vi "rszvl_core_global.vi"() -> ()   [LabVIEW 2014] (continued)
 on the Y axis, the entered numerical values are dimensionless.\n\nAvailable Repeated Capabilities:\nNone\n\nRemote-control command(s):\nCALCulate:STATistics:SCALe:Y:UPPer", "Flags"={"OPC Wait"=FALSE, "Dont check status"=FALSE, "*WAI"=FALSE}, "Check Status Callback"=""}, {"Level"=3, "Descriptive Name"="Signal Statistic Adjust Settings", "Class Only"=FALSE, "Data Type"=4, "Access"=1, "Identifier"="RSZVL_ATTR_MEAS_STAT_ADJ", "Range Table"="", "Command"="CALC:STAT:SCAL:AUTO ONCE", "Read Callback"="", "Write Callback"="", "Range Callback"="", "Check Callback"="", "Rngtable Callback"="", "Coerce Callback"="", "User Callback"="", "Supported Models"="", "Instrument Options"="", "Repeated Capabilities"="", "Restricted Repeated Capabilities"="", "Help"="This attribute optimizes the level setting of the instrument depending on the measured peak power, in order to obtain maximum instrument sensitivity.\nTo obtain maximum resolution, the level range is set as a function of the measured spacing between peak power and the minimum power for the APD measurement and of the spacing between peak power and mean power for the CCDF measurement. In addition, the probability scale for the number of test points is adapted.\n\nAvailable Repeated Capabilities:\nNone\n\nRemote-control command(s):\nCALCulate:STATistics:SCALe:AUTO ONCE", "Flags"={"OPC Wait"=TRUE, "Dont check status"=FALSE, "*WAI"=FALSE}, "Check Status Callback"=""}, {"Level"=3, "Descriptive Name"="Signal Statistic Default Setting", "Class Only"=FALSE, "Data Type"=4, "Access"=1, "Identifier"="RSZVL_ATTR_MEAS_STAT_PRESET", "Range Table"="", "Command"="CALC:STAT:PRES", "Read Callback"="", "Write Callback"="", "Range Callback"="", "Check Callback"="", "Rngtable Callback"="", "Coerce Callback"="", "User Callback"="", "Supported Models"="", "Instrument Options"="", "Repeated Capabilities"="", "Restricted Repeated Capabilities"="", "Help"="This attribute resets the scaling of the X and Y axes in a statistical measurement. The following values are set:\nX axis ref level: -20 dBm\nX axis range APD: 100 dB\nX axis range CCDF: 20 dB\nY axis upper limit: 1.0\nY axis lower limit: 1E-6\n\nAvailable Repeated Capabilities:\nNone\n\nRemote-control command(s):\nCALCulate:STATistics:PRESet", "Flags"={"OPC Wait"=FALSE, "Dont check status"=FALSE, "*WAI"=FALSE}, "Check Status Callback"=""}, {"Level"=3, "Descriptive Name"="Signal Statistic Result", "Class Only"=FALSE, "Data Type"=1, "Access"=0, "Identifier"="RSZVL_ATTR_STAT_RESULT", "Range Table"="", "Command"="CALC:STAT:RES{Trace}? {StatisticMeasType}", "Read Callback"="", "Write Callback"="", "Range Callback"="", "Check Callback"="", "Rngtable Callback"="", "Coerce Callback"="", "User Callback"="", "Supported Models"="", "Instrument Options"="", "Repeated Capabilities"="", "Restricted Repeated Capabilities"="", "Help"="This attribute reads out the results of statistical measurements of a recorded trace.\n\nAvailable Repeated Capabilities:\nTrace: TR1,TR2,TR3,TR4,TR5,TR6,TR7,TR8,TR9,TR10,TR11,TR12,TR13,TR14,TR15,TR16,TR17,TR18,TR19,TR20\r\nStatisticMeasType: StatMean,StatPeak,StatCrestFactor\r\n\nRemote-control command(s):\nCALCulate:STATistics:RESult<1 to 3>? MEAN | PEAK | CFACtor", "Flags"={"OPC Wait"=FALSE, "Dont check status"=FALSE, "*WAI"=FALSE}, "Check Status Callback"=""}, {"Level"=2, "Descriptive Name"="Modulation Depth", "Class Only"=TRUE, "Data Type"=0, "Access"=0, "Identifier"="", "Range Table"="", "Command"="", "Read Callback"="", "Write Callback"="", "Range Callback"="", "Check Callback"="", "Rngtable Callback"="", "Coerce Callback"="", "User Callback"="", "Supported Models"="", "Instrument Options"="", "Repeated Capabilities"="", "Restricted Repeated Capabilities"="", "Help"="Modulation Depth measurement configuration and results.", "Flags"={"OPC Wait"=FALSE, "Dont check status"=FALSE, "*WAI"=FALSE}, "Check Status Callback"=""}, {"Level"=3, "Descriptive Name"="Modulation Depth State", "Class Only"=FALSE, "Data Type"=3, "Access"=2, "Identifier"="RSZVL_ATTR_MEAS_MDEPTH_STATE", "Range Table"="", "Command"="CALC:MARK:FUNC:MDEP", "Read Callback"="", "Write Callback"="", "Range Callback"="", "Check Callback"="", "Rngtable Callback"="", "Coerce Callback"="", "User Callback"="", "Supported Models"="", "Instrument Options"="", "Repeated Capabilities"="", "Restricted Repeated Capabilities"="", "Help"="This attribute switches on the measurement of the AM modulation depth. An AM-modulated carrier is required on the screen for correct operation. If necessary, marker 1 is previously activated and set to the largest signal available.\nThe level value of marker 1 is regarded as the carrier level. On activating the function, marker 2 and marker 3 are automatically set as delta markers symetrically to the carrier to the adjacent maxima of the trace.\nIf the position of delta marker 2 is changed, delta marker 3 is moved symetrically with respect to the reference marker (marker 1). If the position of delta marker 3 is changed, fine adjustment can be performed independently of delta marker 2.\nInstrument calculates the power at the marker positions from the measured levels.\nThe AM modulation depth is calculated from the ratio of power values at the reference marker and the delta markers. If the two AM sidebands differ in power, the average value of the two power values is used for calculating the AM modulation depth.\n\nAvailable Repeated Capabilities:\nNone\n\nRemote-control command(s):\nCALCulate<1|2>:MARKer<1 to 4>:FUNCtion:MDEPth:[:STATe]", "Flags"={"OPC Wait"=FALSE, "Dont check status"=FALSE, "*WAI"=FALSE}, "Check Status Callback"=""}, {"Level"=3, "Descriptive Name"="Modulation Depth Result", "Class Only"=FALSE, "Data Type"=1, "Access"=0, "Identifier"="RSZVL_ATTR_MEAS_MDEPTH_RESULT", "Range Table"="", "Command"="CALC:MARK:FUNC:MDEP:RES?", "Read Callback"="", "Write Callback"="", "Range Callback"="", "Check Callback"="", "Rngtable Callback"="", "Coerce Callback"="", "User Callback"="", "Supported Models"="", "Instrument Options"="", "Repeated Capabilities"="", "Restricted Repeated Capabilities"="", "Help"="This attribute queries the AM modulation depth.\nA complete sweep with synchronization to sweep end must be performed between switching on the function and querying the measured value to obtain a valid query result. This is only possible in single sweep mode.\n\nAvailable Repeated Capabilities:\nNone\n\nRemote-control command(s):\nCALCulate<1|2>:MARKer<1 to 4>:FUNCtion:MDEPth:RESult?", "Flags"={"OPC Wait"=FALSE, "Dont check status"=FALSE, "*WAI"=FALSE}, "Check Status Callback"=""}, {"Level"=3, "Descriptive Name"="Modulation Depth Search", "Class Only"=FALSE, "Data Type"=4, "Access"=1, "Identifier"="RSZVL_ATTR_MEAS_MDEPTH_SEARCH", "Range Table"="", "Command"="CALC:MARK:FUNC:MDEP:SEAR ONCE", "Read Callback"="", "Write Callback"="", "Range Callback"="", "Check Callback"="", "Rngtable Callback"="", "Coerce Callback"="", "User Callback"="", "Supported Models"="", "Instrument Options"="", "Repeated Capabilities"="", "Restricted Repeated Capabilities"="", "Help"="This command starts the search of the signals required for the modulation depth measurement.\n\nAvailable Repeated Capabilities:\nNone\n\nRemote-control command(s):\nCALCulate<1|2>:MARKer<1...4>:FUNCtion:MDEPth:SEARchsignal", "Flags"={"OPC Wait"=FALSE, "Dont check status"=FALSE, "*WAI"=FALSE}, "Check Status Callback"=""}, {"Level"=2, "Descriptive Name"="Third Order Intercept", "Class Only"=TRUE, "Data Type"=0, "Access"=0, "Identifier"="", "Range Table"="", "Command"="", "Read Callback"="", "Write Callback"="", "Range Callback"="", "Check Callback"="", "Rngtable Callback"="", "Coerce Callback"="", "User Callback"="", "Supported Models"="", "Instrument Options"="", "Repeated Capabilities"="", "Restricted Repeated Capabilities"="", "Help"="Third Order Intercept measurement configuration and results.", "Flags"={"OPC Wait"=FALSE, "Dont check status"=FALSE, "*WAI"=FALSE}, "Check Status Callback"=""}, {"Level"=3, "Descriptive Name"="TOI State", "Class Only"=FALSE, "Data Type"=3, "Access"=2, "Identifier"="RSZVL_ATTR_MEAS_TOI_STATE", "Range Table"="", "Command"="CALC:MARK:FUNC:TOI", "Read Callback"="", "Write Callback"="", "Range Callback"="", "Check Callback"="", "Rngtable Callback"="", "Coerce Callback"="", "User Callback"="", "Supported Models"="", "Instrument Options"="", "Repeated Capabilities"="", "Restricted Repeated Capabilities"="", "Help"="This attribute initiates the measurement of the third-order intercept point.\nA two-tone signal with equal carrier levels is expected at the RF input of the instrument. Marker 1 and marker 2 (both normal markers) are set to the maximum of the two signals. Delta marker 3 and delta marker 4 are positioned to the intermodulation products. The delta markers can be modified sperately afterwards.\nThe third-order intercept is calculated from the level spacing between the normal markers and the delta markers.\n\nAvailable Repeated Capabilities:\nNone\n\nRemote-control command(s):\nCALCulate<1|2>:MARKer<1 to 4>:FUNCtion:TOI[:STATe] ON | OFF", "Flags"={"OPC Wait"=FALSE, "Dont check status"=FALSE, "*WAI"=FALSE}, "Check Status Callback"=""}, {"Level"=3, "Descriptive Name"="TOI Result", "Class Only"=FALSE, "Data Type"=1, "Access"=0, "Identifier"="RSZVL_ATTR_MEAS_TOI_RESULT", "Range Table"="", "Command"="CALC:MARK:FUNC:TOI:RES?", "Read Callback"="", "Write Callback"="", "Range Callback"="", "Check Callback"="", "Rngtable Callback"="", "Coerce Callback"="", "User Callback"="", "Supported Models"="", "Instrument Options"="", "Repeated Capabilities"="", "Restricted Repeated Capabilities"="", "Help"="This atttribute queries the third-order intercept point measurement.\nA complete sweep with synchronization to sweep end must be performed between switching on the function and querying the measured value to obtain a valid query result. This is only possible in single sweep mode.\n\nAvailable Repeated Capabilities:\nNone\n\nRemote-control command(s):\nCALCulate<1|2>:MARKer<1 to 4>:FUNCtion:TOI:RESult?", "Flags"={"OPC Wait"=FALSE, "Dont check status"=FALSE, "*WAI"=FALSE}, "Check Status Callback"=""}, {"Level"=3, "Descriptive Name"="TOI Search Signal", "Class Only"=FALSE, "Data Type"=4, "Access"=1, "Identifier"="RSZVL_ATTR_MEAS_TOI_SEARCH", "Range Table"="", "Command"="CALC:MARK{Marker}:FUNC:TOI:SEAR ONCE", "Read Callback"="", "Write Callback"="", "Range Callback"="", "Check Callback"="", "Rngtable Callback"="", "Coerce Callback"="", "User Callback"="", "Supported Models"="", "Instrument Options"="", "Repeated Capabilities"="", "Restricted Repeated Capabilities"="", "Help"="This command starts the search of the signals required for the third order intercept measurement.\n\nAvailable Repeated Capabilities:\nMarker: M1,M2,M3,M4\r\n\nRemote-control command(s):\nCALCulate<1|2>:MARKer<1...4>:FUNCtion:TOI:SEARchsignal", "Flags"={"OPC Wait"=FALSE, "Dont check status"=FALSE, "*WAI"=FALSE}, "Check Status Callback"=""}, {"Level"=2, "Descriptive Name"="Harmonic Distortion", "Class Only"=TRUE, "Data Type"=0, "Access"=0, "Identifier"="", "Range Table"="", "Command"="", "Read Callback"="", "Write Callback"="", "Range Callback"="", "Check Callback"="", "Rngtable Callback"="", "Coerce Callback"="", "User Callback"="", "Supported Models"="", "Instrument Options"="", "Repeated Capabilities"="", "Restricted Repeated Capabilities"="", "Help"="Harmonic Distortion measurement configuration and results.", "Flags"={"OPC Wait"=FALSE, "Dont check status"=FALSE, "*WAI"=FALSE}, "Check Status Callback"=""}, {"Level"=3, "Descriptive Name"="Harmonic Distortion State", "Class Only"=FALSE, "Data Type"=3, "Access"=2, "Identifier"="RSZVL_ATTR_MEAS_HDIST_STATE", "Range Table"="", "Command"="CALC:MARK:FUNC:HARM", "Read Callback"="", "Write Callback"="", "Range Callback"="", "Check Callback"="", "Rngtable Callback"="", "Coerce Callback"="", "User Callback"="", "Supported Models"="", "Instrument Options"="", "Repeated Capabilities"="", "Restricted Repeated Capabilities"="", "Help"="This attribute switches on or off the measurement of the harmonics of a carrier signal. The carrier signal is the first harmonic. The function is independent of the marker selection. It is only available in the frequency domain (span > 0).\nIf the measurement is started in the frequency domain (span > 0), the last span will define the search range for the first harmonic. The level for the first harmonic will also be calculated in the frequency domain. However, the measurement can also be started in the time domain (span = 0), in which case the center frequency and the level used will remain unchanged.\n\nAvailable Repeated Capabilities:\nNone\n\nRemote-control command(s):\nCALCulate<1|2>:MARKer<1 to 4>:FUNCtion:HARMonics[:STATe] ON | OFF", "Flags"={"OPC Wait"=TRUE, "Dont check status"=FALSE, "*WAI"=FALSE}, "Check Status Callback"=""}, {"Level"=3, "Descriptive Name"="Harmonic Distortion No Of Harmonics", "Class Only"=FALSE, "Data Type"=0, "Access"=2, "Identifier"="RSZVL_ATTR_MEAS_HDIST_NOOFHARM", "Range Table"="rszvl_rngMeasHDISTNharm", "Command"="CALC:MARK:FUNC:HARM:NHAR", "Read Callback"="", "Write Callback"="", "Range Callback"="", "Check Callback"="", "Rngtable Callback"="", "Coerce Callback"="", "User Callback"="", "Supported Models"="", "Instrument Options"="", "Repeated Capabilities"="", "Restricted Repeated Capabilities"="", "Help"="This attribute defines the number of harmonics of a carrier signal to be measured. The function is independent of the marker selection.\n\nAvailable Repeated Capabilities:\nNone\n\nRemote-control command(s):\nCALCulate<1|2>:MARKer<1 to 4>:FUNCtion:HARMonics:NHARmonics", "Flags"={"OPC Wait"=FALSE, "Dont check status"=FALSE, "*WAI"=FALSE}, "Check Status Callback"=""}, {"Level"=3, "Descriptive Name"="Harmonic Distortion RBW Auto", "Class Only"=FALSE, "Data Type"=3, "Access"=2, "Identifier"="RSZVL_ATTR_MEAS_HDIST_RBWAUTO", "Range Table"="", "Command"="CALC:MARK:FUNC:HARM:BAND:AUTO", "Read Callback"="", "Write Callback"="", "Range Callback"="", "Check Callback"="", "Rngtable Callback"="", "Coerce Callback"="", "User Callback"="", "Supported Models"="", "Instrument Options"="", "Repeated Capabilities"="", "Restricted Repeated Capabilities"="", "Help"="This attribute specifies whether the resolution bandwidth of the 2nd to the nth harmonic should be identical to the bandwidth of the first harmonic (OFF) or to the next largest bandwidth (corresponding to the harmonic) of the multiple of the bandwidth of the first harmonic (ON).\n\nAvailable Repeated Capabilities:\nNone\n\nRemote-control command(s):\nCALCulate<1|2>:MARKer<1 to 4>:FUNCtion:HARMonics:BANDwidth:AUTO ON | OFF", "Flags"={"OPC Wait"=FALSE, "Dont check status"=FALSE, "*WAI"=FALSE}, "Check Status Callback"=""}, {"Level"=3, "Descriptive Name"="Harmonic Distortion Adjust Settings", "Class Only"=FALSE, "Data Type"=4, "Access"=1, "Identifier"="RSZVL_ATTR_MEAS_HDIST_PRESET", "Range Table"="", "Command"="CALC:MARK:FUNC:HARM:PRES", "Read Callback"="", "Write Callback"="", "Range Callback"="", "Check Callback"="", "Rngtable Callback"="", "Coerce Callback"="", "User Callback"="", "Supported Models"="", "Instrument Options"="", "Repeated Capabilities"="", "Restricted Repeated Capabilities"="", "Help"="This attribute optimizes the device settings depending on the mode in which the harmonic measurement was started:\nIf the harmonic measurement was started in the frequency domain (span > 0), the frequency and the level of the first harmonic are calculated, from which the measurement list is set up.\nIf the measurement was started in the time domain (span = 0), the frequency of the first harmonic is not changed. The level, however, is not calculated.\nThe function is independent of the marker selection.\n\nAvailable Repeated Capabilities:\nNone\n\nRemote-control command(s):\nCALCulate<1|2>:MARKer<1 to 4>:FUNCtion:HARMonics:PRESet", "Flags"={"OPC Wait"=TRUE, "Dont check status"=FALSE, "*WAI"=FALSE}, "Check Status Callback"=""}, {"Level"=2, "Descriptive Name"="Burst Power", "Class Only"=TRUE, "Data Type"=0, "Access"=0, "Identifier"="", "Range Table"="", "Command"="", "Read Callback"="", "Write Callback"="", "Range Callback"="", "Check Callback"="", "Rngtable Callback"="", "Coerce Callback"="", "User Callback"="", "Supported Models"="", "Instrument Options"="", "Repeated Capabilities"="", "Restricted Repeated Capabilities"="", "Help"="Burst Power measurement configuration and results.", "Flags"={"OPC Wait"=FALSE, "Dont check status"=FALSE, "*WAI"=FALSE}, "Check Status Callback"=""}, {"Level"=3, "Descriptive Name"="Burst Power Minimum Value", "Class Only"=FALSE, "Data Type"=1, "Access"=0, "Identifier"="RSZVL_ATTR_MPOW_MIN", "Range Table"="", "Command"="*WAI;SENS:MPOW:RES:MIN?", "Read Callback"="", "Write Callback"="", "Range Callback"="", "Check Callback"="", "Rngtable Callback"="", "Coerce Callback"="", "User Callback"="", "Supported Models"="", "Instrument Options"="", "Repeated Capabilities"="", "Restricted Repeated Capabilities"="", "Help"="Thsi attribute queries the minimum power value in a multiple burst power measurement.\n\nAvailable Repeated Capabilities:\nNone\n\nRemote-control command(s):\n[SENSe<1|2>:]MPOWer:RESult:MIN?", "Flags"={"OPC Wait"=FALSE, "Dont check status"=FALSE, "*WAI"=FALSE}, "Check Status Callback"=""}, {"Level"=3, "Descriptive Name"="Burst Power Filter Type", "Class Only"=FALSE, "Data Type"=0, "Access"=2, "Identifier"="RSZVL_ATTR_MPOW_FTYPE", "Range Table"="rszvl_rngMpowFiltType", "Command"="SENS:MPOW:FTYP", "Read Callback"="", "Write Callback"="", "Range Callback"="", "Check Callback"="", "Rngtable Callback"="", "Coerce Callback"="", "User Callback"="", "Supported Models"="", "Instrument Options"="", "Repeated Capabilities"="", "Restricted Repeated Capabilities"="", "Help"="This attribute defines the filter type for the measurement.\n\nAvailable Repeated Capabilities:\nNone\n\nRemote-control command(s):\n[SENSe<1|2>:]MPOWer:FTYPe", "Flags"={"OPC Wait"=FALSE, "Dont check status"=FALSE, "*WAI"=FALSE}, "Check Status Callback"=""}, {"Level"=2, "Descriptive Name"="IQ Measurement", "Class Only"=TRUE, "Data Type"=0, "Access"=0, "Identifier"="", "Range Table"="", "Command"="", "Read Callback"="", "Write Callback"="", "Range Callback"="", "Check Callback"="", "Rngtable Callback"="", "Coerce Callback"="", "User Callback"="", "Supported Models"="", "Instrument Options"="", "Repeated Capabilities"="", "Restricted Repeated Capabilities"="", "Help"="IQ  measurement configuration and results.", "Flags"={"OPC Wait"=FALSE, "Dont check status"=FALSE, "*WAI"=FALSE}, "Check Status Callback"=""}, {"Level"=3, "Descriptive Name"="IQ Sample Rate", "Class Only"=FALSE, "Data Type"=1, "Access"=2, "Identifier"="RSZVL_ATTR_IQ_SAMPLE_RATE", "Range Table"="rszvl_rngIQSRate", "Command"="TRAC:IQ:SRAT", "Read Callback"="", "Write Callback"="", "Range Callback"="", "Check Callback"="", "Rngtable Callback"="", "Coerce Callback"="", "User Callback"="", "Supported Models"="", "Instrument Options"="", "Repeated Capabilities"="", "Restricted Repeated Capabilities"="", "Help"="This attribute sets the sampling rate for the I/Q data acquisition. Thus the sample rate can be modified without affecting the other settings.\n\nNote:\n(1) Value range: 15.625 kHz, 31.25 kHz, 62.5 kHz,\n125 kHz, 250 kHz, 500 kHz,\n1 MHz, 2 MHz, 4 MHz, 8 MHz, 16 MHz, 32 MHz\n\nValue range: 10.0 kHz to 81.6 MHz sampling rates require a bandwidth of 50 MHz, set with the TRAC:IQ:SET\ncommand.\n\n(2) If <filter type> = CFILter, the sample rate is determined by the selected filter bandwidth. In\nthis case, the currently set sample rate can be determined using the query command.\nEntering a value causes an execution error if <filter type> = CFILter.\n\nAvailable Repeated Capabilities:\nNone\n\nRemote-control command(s):\nTRACe<1|2>:IQ:SRATe", "Flags"={"OPC Wait"=FALSE, "Dont check status"=FALSE, "*WAI"=FALSE}, "Check Status Callback"=""}, {"Level"=3, "Descriptive Name"="IQ Data Acquisition", "Class Only"=FALSE, "Data Type"=3, "Access"=2, "Identifier"="RSZVL_ATTR_IQ_DATA_STATE", "Range Table"="", "Command"="TRAC:IQ", "Read Callback"="", "Write Callback"="", "Range Callback"="", "Check Callback"="", "Rngtable Callback"="", "Coerce Callback"="", "User Callback"="", "Supported Models"="", "Instrument Options"="", "Repeated Capabilities"="", "Restricted Repeated Capabilities"="", "Help"="This attribute switches the I/Q data acquisition on or off.\n\nNote:\n(1) The I/Q data acquisition is not compatible with other measurement functions. Therefore all other measurement functions will be switched off as soon as the I/Q measurement function is switched on. Additionally a trace display is not possible in this operating mode. Therefore all traces are set to BLANK. Finally split screen operation will automatically be stopped.\n\nAvailable Repeated Capabilities:\nNone\n\nRemote-control command(s):\nTRACe<1|2>:IQ[:STATe] ON | OFF", "Flags"={"OPC Wait"=FALSE, "Dont check status"=FALSE, "*WAI"=FALSE}, "Check Status Callback"=""}, {"Level"=3, "Descriptive Name"="IQ Data Averaging State", "Class Only"=FALSE, "Data Type"=3, "Access"=2, "Identifier"="RSZVL_ATTR_IQ_DATA_AVER_STATE", "Range Table"="", "Command"="TRAC:IQ:AVER", "Read Callback"="", "Write Callback"="", "Range Callback"="", "Check Callback"="", "Rngtable Callback"="", "Coerce Callback"="", "User Callback"="", "Supported Models"="", "Instrument Options"="", "Repeated Capabilities"="", "Restricted Repeated Capabilities"="", "Help"="This attribute enables averaging of the recorded I/Q data provided that I/Q data acquisition was previously enabled with TRACe<1|2>:IQ[:STATe].\n\nAvailable Repeated Capabilities:\nNone\n\nRemote-control command(s):\nTRACe<1|2>:IQ:AVERage[:STATe]", "Flags"={"OPC Wait"=FALSE, "Dont check status"=FALSE, "*WAI"=FALSE}, "Check Status Callback"=""}, {"Level"=3, "Descriptive Name"="IQ Data Averaging Count", "Class Only"=FALSE, "Data Type"=0, "Access"=2, "Identifier"="RSZVL_ATTR_IQ_DATA_AVER_COUNT", "Range Table"="rszvl_rngSweepCount", "Command"="TRAC:IQ:AVER:COUN", "Read Callback"="", "Write Callback"="", "Range Callback"="", "Check Callback"="", "Rngtable Callback"="", "Coerce Callback"="", "User Callback"="", "Supported Models"="", "Instrument Options"="", "Repeated Capabilities"="", "Restricted Repeated Capabilities"="", "Help"="This attribute defines the number of I/Q data sets that are to serve as a basis for averaging.\n\nAvailable Repeated Capabilities:\nNone\n\nRemote-control command(s):\nTRACe<1|2>:IQ:AVERage:COUNt", "Flags"={"OPC Wait"=FALSE, "Dont check status"=FALSE, "*WAI"=FALSE}, "Check Status Callback"=""}, {"Level"=1, "Descriptive Name"="Miscellaneous Attributes", "Class Only"=TRUE, "Data Type"=0, "Access"=0, "Identifier"="", "Range Table"="", "Command"="", "Read Callback"="", "Write Callback"="", "Range Callback"="", "Check Callback"="", "Rngtable Callback"="", "Coerce Callback"="", "User Callback"="", "Supported Models"="", "Instrument Options"="", "Repeated Capabilities"="", "Restricted Repeated Capabilities"="", "Help"="(1) ID Query Response:\nReturns the ID Query response string. The instrument driver gets the value of this attribute when you pass VI_TRUE for the ID Query parameter to the rszvl_init or rszvl_InitWithOptions function.", "Flags"={"OPC Wait"=FALSE, "Dont check status"=FALSE, "*WAI"=FALSE}, "Check Status Callback"=""}, {"Level"=2, "Descriptive Name"="ID Query Response", "Class Only"=FALSE, "Data Type"=2, "Access"=2, "Identifier"="RSZVL_ATTR_ID_QUERY_RESPONSE", "Range Table"="", "Command"="", "Read Callback"="", "Write Callback"="", "Range Callback"="", "Check Callback"="", "Rngtable Callback"="", "Coerce Callback"="", "User Callback"="", "Supported Models"="", "Instrument Options"="", "Repeated Capabilities"="", "Restricted Repeated Capabilities"="", "Help"="Returns the ID Query response string. The instrument driver gets the value of this attribute when you pass VI_TRUE for the ID Query parameter to the rszvl_init or rszvl_InitWithOptions function.\n\nAvailable Repeated Capabilities:\nNone\n\nRemote-control command(s):\n", "Flags"={"OPC Wait"=FALSE, "Dont check status"=TRUE, "*WAI"=FALSE}, "Check Status Callback"=""}, {"Level"=1, "Descriptive Name"="Service", "Class Only"=TRUE, "Data Type"=0, "Access"=0, "Identifier"="", "Range Table"="", "Command"="", "Read Callback"="", "Write Callback"="", "Range Callback"="", "Check Callback"="", "Rngtable Callback"="", "Coerce Callback"="", "User Callback"="", "Supported Models"="", "Instrument Options"="", "Repeated Capabilities"="", "Restricted Repeated Capabilities"="", "Help"="(1) Service Input Source:\nThis attribute toggles between the RF input on the front panel and the internal 128-MHz reference signal. The level of the 128-MHz signals can be selected by attribute RSZVL_ATTR_SERVICE_INPUT_LEVEL.\n\n(2) Service Input Comb Frequency:\nThis attribute sets the comb generator frequency.\n\n(3) Service Noise Source:\nThis attribute switches the 28-V supply of the noise source at the rear panel on or off.\n\n(4) Self Test Results:\nThis attribute reads the results of the selftest out of the instrument. The lines of the result table are output as string data separated by commas.\n\n(5) Self Test:\nThis attribute initiates the selftest of the instrument and outputs an error code in decimal form.\n0 - passed\n1 - failed", "Flags"={"OPC Wait"=FALSE, "Dont check status"=FALSE, "*WAI"=FALSE}, "Check Status Callback"=""}, {"Level"=2, "Descriptive Name"="Service Input Source", "Class Only"=FALSE, "Data Type"=0, "Access"=2, "Identifier"="RSZVL_ATTR_SERVICE_INPUT_SOURCE", "Range Table"="rszvl_rngServiceInput", "Command"="DIAG:SERV:INP", "Read Callback"="", "Write Callback"="", "Range Callback"="", "Check Callback"="", "Rngtable Callback"="", "Coerce Callback"="", "User Callback"="", "Supported Models"="", "Instrument Options"="", "Repeated Capabilities"="", "Restricted Repeated Capabilities"="", "Help"="This attribute toggles between the RF input on the front panel and the internal 128-MHz reference signal. The level of the 128-MHz signals can be selected by attribute RSZVL_ATTR_SERVICE_INPUT_LEVEL.\n\nAvailable Repeated Capabilities:\nNone\n\nRemote-control command(s):\nDIAGnostic<1|2>:SERVice:INPut[:SELect] CALibration | RF | TG", "Flags"={"OPC Wait"=FALSE, "Dont check status"=FALSE, "*WAI"=FALSE}, "Check Status Callback"=""}, {"Level"=2, "Descriptive Name"="Service Input Comb Frequency", "Class Only"=FALSE, "Data Type"=0, "Access"=2, "Identifier"="RSZVL_ATTR_SERVICE_INPUT_COMB_FREQUENCY", "Range Table"="rszvl_rngServiceCombFrequency", "Command"="DIAG:SERV:INP:PULS:PRAT", "Read Callback"="", "Write Callback"="", "Range Callback"="", "Check Callback"="", "Rngtable Callback"="", "Coerce Callback"="", "User Callback"="", "Supported Models"="", "Instrument Options"="", "Repeated Capabilities"="", "Restricted Repeated Capabilities"="", "Help"="This attribute sets the comb generator frequency.\n\nAvailable Repeated Capabilities:\nNone\n\nRemote-control command(s):\nDIAGnostic<1|2>:SERVice:INPut:PULSed:PRATe", "Flags"={"OPC Wait"=FALSE, "Dont check status"=FALSE, "*WAI"=FALSE}, "Check Status Callback"=""}, {"Level"=2, "Descriptive Name"="Service Noise Source", "Class Only"=FALSE, "Data Type"=3, "Access"=2, "Identifier"="RSZVL_ATTR_SERVICE_NOISE_SOURCE", "Range Table"="", "Command"="DIAG:SERV:NSO", "Read Callback"="", "Write Callback"="", "Range Callback"="", "Check Callback"="", "Rngtable Callback"="", "Coerce Callback"="", "User Callback"="", "Supported Models"="", "Instrument Options"="", "Repeated Capabilities"="", "Restricted Repeated Capabilities"="", "Help"="This attribute switches the 28-V supply of the noise source at the rear panel on or off.\n\nAvailable Repeated Capabilities:\nNone\n\nRemote-control command(s):\nDIAGnostic<1|2>:SERVice:NSOurce ON | OFF", "Flags"={"OPC Wait"=FALSE, "Dont check status"=FALSE, "*WAI"=FALSE}, "Check Status Callback"=""}, {"Level"=2, "Descriptive Name"="Self Test Results", "Class Only"=FALSE, "Data Type"=2, "Access"=0, "Identifier"="RSZVL_ATTR_SERVICE_STEST_RESULTS", "Range Table"="", "Command"="DIAG:SERV:STES:RES?", "Read Callback"="", "Write Callback"="", "Range Callback"="", "Check Callback"="", "Rngtable Callback"="", "Coerce Callback"="", "User Callback"="", "Supported Models"="", "Instrument Options"="", "Repeated Capabilities"="", "Restricted Repeated Capabilities"="", "Help"="This attribute reads the results of the selftest out of the instrument. The lines of the result table are output as string data separated by commas.\n\nAvailable Repeated Capabilities:\nNone\n\nRemote-control command(s):\nDIAGnostic<1|2>:SERVice:STESt:RESult?", "Flags"={"OPC Wait"=FALSE, "Dont check status"=FALSE, "*WAI"=FALSE}, "Check Status Callback"=""}, {"Level"=2, "Descriptive Name"="Self Test", "Class Only"=FALSE, "Data Type"=0, "Access"=0, "Identifier"="RSZVL_ATTR_SERVICE_STEST", "Range Table"="", "Command"="*TST?", "Read Callback"="", "Write Callback"="", "Range Callback"="", "Check Callback"="", "Rngtable Callback"="", "Coerce Callback"="", "User Callback"="", "Supported Models"="", "Instrument Options"="", "Repeated Capabilities"="", "Restricted Repeated Capabilities"="", "Help"="This attribute initiates the selftest of the instrument and outputs an error code in decimal form.\n0 - passed\n1 - failed\n\nAvailable Repeated Capabilities:\nNone\n\nRemote-control command(s):\n*TST?", "Flags"={"OPC Wait"=TRUE, "Dont check status"=FALSE, "*WAI"=FALSE}, "Check Status Callback"=""}, {"Level"=1, "Descriptive Name"="File", "Class Only"=TRUE, "Data Type"=0, "Access"=0, "Identifier"="", "Range Table"="", "Command"="", "Read Callback"="", "Write Callback"="", "Range Callback"="", "Check Callback"="", "Rngtable Callback"="", "Coerce Callback"="", "User Callback"="", "Supported Models"="", "Instrument Options"="", "Repeated Capabilities"="", "Restricted Repeated Capabilities"="", "Help"="(1) File Recall:\nThis attribute loads device settings from files.The contents of the file are loaded and set as the new device state. The device automatically recognizes the files that are required for the whole setup.\n\n(2) File Startup Recall:\nThis attribute defines which device setting is automatically loaded after the device is switched on. The contents of the file are read after switching on the device and used to define the new device state. The file name includes indication of the path and may also include the drive. The path name complies with DOS conventions.\n\n(3) File Save:\nThis attribute stores the current device settings in a series of files which have the indicated file name, but different extensions. The file name includes indication of the path and may also include the drive name. The path name complies with DOS conventions. The numeric suffix in STORe<1|2> is irrelevant with this command. A list of the extensions used is contained under MMEMory:LOAD:STATe.\n\n(4) File Data Set Clear:\nThis command deletes the instrument setting selected by <file_name>. All associated files on the mass memory storage are cleared. A list of the extensions used is included under MMEMory:LOAD:STATe. The file name includes indication of the path and may also include the drive. The path name complies with DOS conventions.\n\n(5) File Data Set Clear All:\nThis attribute deletes all device settings in the current directory.The current directory can be selected with MMEM:CDIR. The default directory is D:.\n\n(6) File Decimal Separator:\nThis attribute defines which decimal separator (decimal point or comma) is to be used for outputting measurement data to the file in ASCII format.\n\n(7) Manager (Class):\nFile management attributes.\n\n(1) File Manager Edit Path:\nThis attribute changes the current directory.\nIn addition to the path name, the indication of the directory may contain the drive name. The path name complies with the DOS conventions.\n\n(2) File Manager Delete:\n\n\n(3) File Manager Make Directory:\nThis attribute creates a new directory. The file name includes indication of the path and may also include the drive name. The path name complies with DOS conventions.\n\n(4) File Manager Edit Path Device:\nThis attribute changes to the drive indicated. The drive may be the internal hard disk D: or the floppy disk drive A:.\n\n(5) File Manager Delete Directory:\nThis attribute deletes the indicated directory. The directory name includes indication of the path and may also include the drive name. The path name complies with DOS conventions.\n\n\n\n(8) Save Recall (Class):\nConfiguration of stored setups.\n\n(1) File Items to Save Recall Select Source Cal Data:\nThis attribute adds the tracking generator calibration data to the list of device settings to be stored/loaded.\n\n(2) File Items to Save Recall Select All Transducers:\nThis attribute includes all transducer factors and sets in the list of data subsets of a device setting to be stored/loaded.\n\n(3) File Items to Save Recall Select HW Settings:\nThis attribute includes the hardware settings in the list of data subsets of a device setting to be stored/loaded. The hardware settings include:\n- current configuration of general device parameters (general setup)\n- current setting of the measurement hardware including markers\n- activated limit lines:\nA data set may include 8 limit lines at maximum. This number includes the activated limit lines and, if available, the de-activated limit lines last used. Therefore the combination of the non-activated restored limit lines depends on the sequence of use with the command MMEM:LOAD.\n- user-defined color setting\n- configuration for the hardcopy output\n- Tracking generator settings (only in conjunction with option External Generator Control B10)\n- Correction data for source calibration (only in conjunction with option External Generator Control B10)\n\n(4) File Items to Save Recall Select Trace:\nThis attribute adds the active traces to the list of data subsets of a save/recall device setting. Active traces are all traces whose state is not blank.\n\n(5) File Items to Save Recall Select Lines:\nThis attribute adds all limit lines (activated and de-activated) to the list of device settings to be\nstored/loaded.\n\n(6) File Items to Save Recall All:\nThis command includes all data subsets in the list device settings to be stored/loaded.\n\n(7) File Items to Save Recall None:\nThis attribute deletes all data subsets from the list of device settings to be stored/loaded.\n\n(8) File Items to Save Recall Default:\nThis attribute sets the default list of device settings to be stored/loaded.The latter includes:\n- current configuration of general device parameters (general setup)\n- current setting of the measurement hardware including markers\n- activated limit lines\n- user-defined color setting\n- configuration for the hardcopy output\n- Tracking generator settings (only in conjunction with option External Generator Control B10)\n- Correction data for source calibration (only in conjunction with option External Generator Control B10)\nTrace data and non-used limit lines are not included.", "Flags"={"OPC Wait"=FALSE, "Dont check status"=FALSE, "*WAI"=FALSE}, "Check Status Callback"=""}, {"Level"=2, "Descriptive Name"="File Recall", "Class Only"=FALSE, "Data Type"=2, "Access"=1, "Identifier"="RSZVL_ATTR_FILE_RECALL", "Range Table"="", "Command"="MMEM:LOAD:STAT", "Read Callback"="", "Write Callback"="rszvl_FileStateSpecialFormat_WriteCallback.vi", "Range Callback"="", "Check Callback"="", "Rngtable Callback"="", "Coerce Callback"="", "User Callback"="", "Supported Models"="", "Instrument Options"="", "Repeated Capabilities"="", "Restricted Repeated Capabilities"="", "Help"="This attribute loads device settings from files.The contents of the file are loaded and set as the new device state. The device automatically recognizes the files that are required for the whole setup.\n\nAvailable Repeated Capabilities:\nNone\n\nRemote-control command(s):\nMMEMory:LOAD:STATe 1,<file_name>", "Flags"={"OPC Wait"=FALSE, "Dont check status"=FALSE, "*WAI"=FALSE}, "Check Status Callback"=""}, {"Level"=2, "Descriptive Name"="File Startup Recall", "Class Only"=FALSE, "Data Type"=2, "Access"=2, "Identifier"="RSZVL_ATTR_FILE_STARTUP_RECALL", "Range Table"="", "Command"="MMEM:LOAD:AUTO", "Read Callback"="", "Write Callback"="rszvl_FileStateSpecialFormat_WriteCallback.vi", "Range Callback"="", "Check Callback"="", "Rngtable Callback"="", "Coerce Callback"="", "User Callback"="", "Supported Models"="", "Instrument Options"="", "Repeated Capabilities"="", "Restricted Repeated Capabilities"="", "Help"="This attribute defines which device setting is automatically loaded after the device is switched on. The contents of the file are read after switching on the device and used to define the new device state. The file name includes indication of the path and may also include the drive. The path name complies with DOS conventions.\n\nAvailable Repeated Capabilities:\nNone\n\nRemote-control command(s):\nMMEMory:LOAD:AUTO 1,<file_name>", "Flags"={"OPC Wait"=FALSE, "Dont check status"=FALSE, "*WAI"=FALSE}, "Check Status Callback"=""}, {"Level"=2, "Descriptive Name"="File Save", "Class Only"=FALSE, "Data Type"=2, "Access"=1, "Identifier"="RSZVL_ATTR_FILE_SAVE", "Range Table"="", "Command"="MMEM:STOR:STAT", "Read Callback"="", "Write Callback"="rszvl_FileStateSpecialFormat_WriteCallback.vi", "Range Callback"="", "Check Callback"="", "Rngtable Callback"="", "Coerce Callback"="", "User Callback"="", "Supported Models"="", "Instrument Options"="", "Repeated Capabilities"="", "Restricted Repeated Capabilities"="", "Help"="This attribute stores the current device settings in a series of files which have the indicated file name, but different extensions. The file name includes indication of the path and may also include the drive name. The path name complies with DOS conventions. The numeric suffix in STORe<1|2> is irrelevant with this command. A list of the extensions used is contained under MMEMory:LOAD:STATe.\n\nAvailable Repeated Capabilities:\nNone\n\nRemote-control command(s):\nMMEMory:STORe<1|2>:STATe 1,<file name>", "Flags"={"OPC Wait"=FALSE, "Dont check status"=FALSE, "*WAI"=FALSE}, "Check Status Callback"=""}, {"Level"=2, "Descriptive Name"="File Data Set Clear", "Class Only"=FALSE, "Data Type"=2, "Access"=1, "Identifier"="RSZVL_ATTR_FILE_DATA_CLEAR", "Range Table"="", "Command"="MMEM:CLE:STAT", "Read Callback"="", "Write Callback"="rszvl_FileStateSpecialFormat_WriteCallback.vi", "Range Callback"="", "Check Callback"="", "Rngtable Callback"="", "Coerce Callback"="", "User Callback"="", "Supported Models"="", "Instrument Options"="", "Repeated Capabilities"="", "Restricted Repeated Capabilities"="", "Help"="This command deletes the instrument setting selected by <file_name>. All associated files on the mass memory storage are cleared. A list of the extensions used is included under MMEMory:LOAD:STATe. The file name includes indication of the path and may also include the drive. The path name complies with DOS conventions.\n\nAvailable Repeated Capabilities:\nNone\n\nRemote-control command(s):\nMMEMory:CLEar:STATe", "Flags"={"OPC Wait"=FALSE, "Dont check status"=FALSE, "*WAI"=FALSE}, "Check Status Callback"=""}, {"Level"=2, "Descriptive Name"="File Data Set Clear All", "Class Only"=FALSE, "Data Type"=4, "Access"=1, "Identifier"="RSZVL_ATTR_FILE_DATA_CLEAR_ALL", "Range Table"="", "Command"="MMEM:CLE:ALL", "Read Callback"="", "Write Callback"="", "Range Callback"="", "Check Callback"="", "Rngtable Callback"="", "Coerce Callback"="", "User Callback"="", "Supported Models"="", "Instrument Options"="", "Repeated Capabilities"="", "Restricted Repeated Capabilities"="", "Help"="This attribute deletes all device settings in the current directory.The current directory can be selected with MMEM:CDIR. The default directory is D:.\n\nAvailable Repeated Capabilities:\nNone\n\nRemote-control command(s):\nMMEMory:CLEar:ALL", "Flags"={"OPC Wait"=FALSE, "Dont check status"=FALSE, 
